vi "PMBus Write Word.vi"(4 "PEC":u8, 5 "Data":u16, 6 "CommandCode":u8, 7 "SlaveAddr":u8, 8 "error in (no error)":errorcluster, 9 "PMBusIndex":i32, 10 "DevIndex":i32, 11 "DevType":i32) -> (0 "error out":errorcluster, 3 "function return":i32)   [LabVIEW 2012, in "ControlPMBus.lvlib"]
doc: "int WINAPI PMBus_WriteWord(int DevType,int DevIndex,int PMBusIndex,unsigned char SlaveAddr,unsigned char CommandCode,unsigned short Data,unsigned char PEC);"
uses:
  ControlPMBus.lvlib
  Ginkgo_Driver.dll
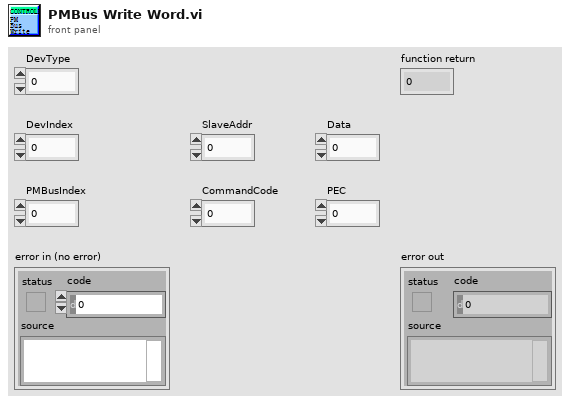
[diagram p1: front panel]
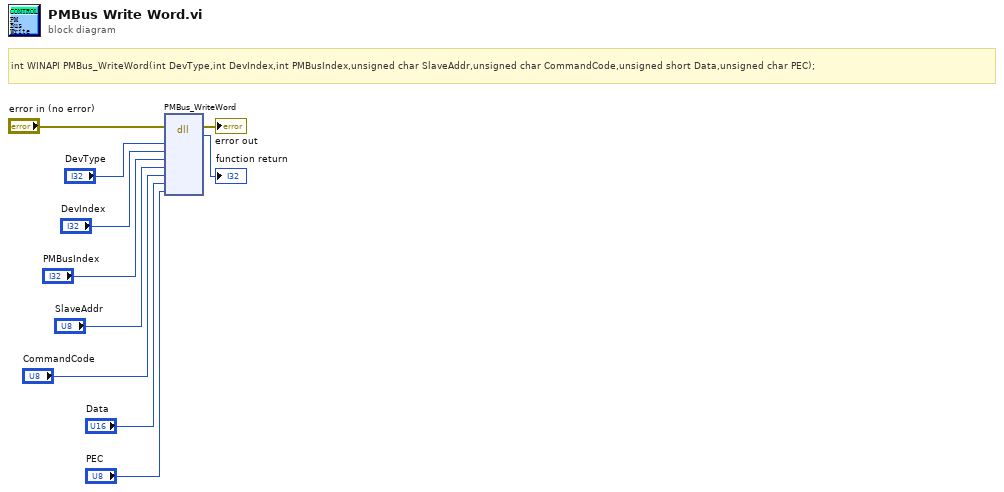
[diagram p0: block diagram]
diagram:
  # "int WINAPI PMBus_WriteWord(int DevType,int DevIndex,int PMBusIndex,unsigned char SlaveAddr,unsigned char CommandCode,unsigned short Data,unsigned char PEC);"
  n1 = dll-call lib="E:/Project/vt_ginkgo/truck/Ginkgo Driver/vs2010/Ginkgo_USB-I2C_API_v2.0.3.0/lib/labview_32bit/ControlPMBus/Ginkgo_Driver.*" fn="PMBus_WriteWord"(error in="error in (no error)", "DevType"="DevType", "DevIndex"="DevIndex", "PMBusIndex"="PMBusIndex", "SlaveAddr"="SlaveAddr", "CommandCode"="CommandCode", "Data"="Data", "PEC"="PEC") -> (error out=→"error out":errorcluster, →"function return":i32)  [unwired: 9 in, 1 out]
